vi "IVIS FRET_Build Overlay.vi"(6 "Color Scale Marker Values":cluster{"Value":dbl, "Color":u32}[](array[cluster]), 8 "Error In":errorcluster, 9 "[DD Pixel Coordinates]":T2[](array[typedef]), 10 "Overlay Values":dbl[](array[numeric]), 11 "Refnum in":T1) -> (0 "Error Out":errorcluster, 3 "Refnum out":T1)   [LabVIEW 2021]
uses:
  Image/Image Point.ctl
  <vilib>/vision/Image Controls.llb/IMAQ Image.ctl
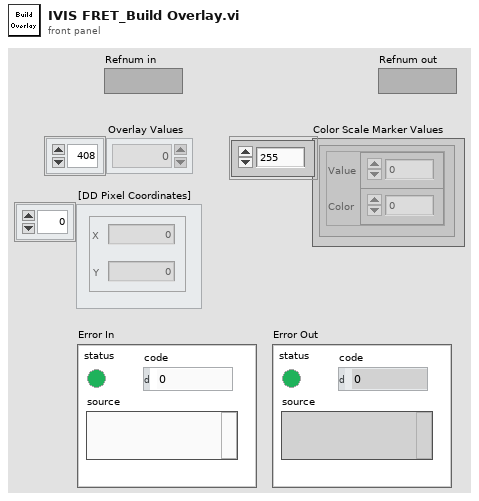
[diagram p1: front panel]
types:
  T1 = typedef "IMAQ Image.ctl" = refnum<image>
  T2 = typedef "Image Point.ctl" = cluster{"X":i32, "Y":i32}
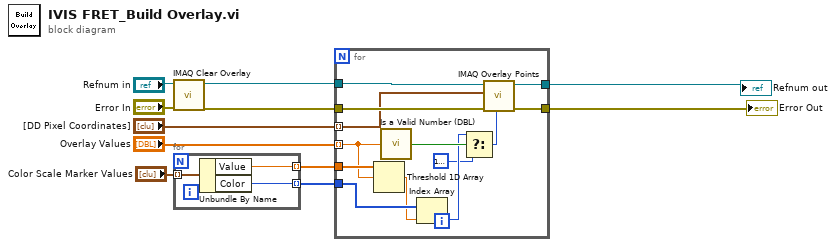
[diagram p0: block diagram]
diagram:
  n1 = call "IMAQ Clear Overlay"("error in (no error)"="Error In", "Image"="Refnum in") -> ("error out"=w8:errorcluster, "Image Out"=w9:T1)  [unwired: 8 in]
  n2 = for {
    tunnel: "Color Scale Marker Values" -> [w14] mode=indexing
    tunnel: [w13] -> w2 mode=indexing
    tunnel: [w12] -> w1 mode=indexing
    n3 = Unbundle By Name(w14) -> ("Value"=w13:dbl, "Color"=w12:u32)
  }
  n4 = for {
    tunnel: w9 -> [w27]
    tunnel: w8 -> [w26]
    tunnel: "Overlay Values" -> [w19] mode=indexing
    tunnel: "[DD Pixel Coordinates]" -> [w25] mode=indexing
    tunnel: [w24] -> w5
    tunnel: [w23] -> w4
    tunnel: w2 -> [w22]
    tunnel: w1 -> [w21]
    n5 = Threshold 1D Array(2:w19, 3:w22) -> (0:w20:dbl)  [unwired: 1 in]
    n6 = call "Is a Valid Number (DBL).vi"("Number"=w19) -> ("Valid Number?"=w18:bool)  [unwired: 8 in]
    n7 = Index Array(array=w21, index=w20) -> (element=w17:u32)
    n8 = Select(t=w17, s=w18, f=u32 16777216 ("Color")) -> (s? t:f=w15:u32)
    n9 = call "IMAQ Overlay Points"("Color"=w15, "error in (no error)"=w26, "Point"=w25, "Image"=w27) -> ("error out"=w23:errorcluster, "Image Out"=w24:T1)  [unwired: 6 in]
  }
  "Error Out" <- w4
  "Refnum out" <- w5
